vi "FirmataConstants.vi"(8 "error in":errorcluster) -> (0 "error out":errorcluster, 2 "FirmataCapabilities":T2 {"Index"."DigitalIndex" step=1 format="D%d"; "Index"."AnalogIndex" min=0.0 step=1.0 format="A%#.0g"})   [LabVIEW 2020, in "FirmataClient.lvlib"]
doc: "Repository for Firmata Protocol Constants\n- https://github.com/firmata/protocol/blob/master/protocol.md"
uses:
  FirmataClient.lvlib
  controls/PinModesListData.ctl
  controls/PinModeData.ctl
  controls/FirmataPinModes.ctl
  controls/FirmataProtocolConstants.ctl
  <vilib>/Utility/miscctls.llb/LVStringsAndValuesArrayTypeDef_U16.ctl
panel:
  in  "Reload Constant?":bool
  out "FimataProtocolConstants":T1 items=["ANALOG_IO_MESSAGE"=224, "DIGITAL_IO_MESSAGE"=144, "REPORT_ANALOG_PIN"=192, "REPORT_DIGITAL_PORT"=208, "START_SYSEX"=240, "END_SYSEX"=247, "SET_PIN_MODE"=244, "SET_DIGITAL_PIN_VALUE"=245, "PROTOCOL_VERSION"=249, "SYSTEM_RESET"=255, "SYSEX.EXTENDED_ID"=0, "SYSEX.RESERVED_USER_COMMANDs"=1, "SYSEX.ANALOG_MAPPING_QUERY"=105, "SYSEX.ANALOG_MAPPING_RESPONSE"=106, "SYSEX.CAPABILITY_QUERY"=107, "SYSEX.CAPABILITY_RESPONSE"=108, "SYSEX.PIN_STATE_QUERY"=109, "SYSEX.PIN_STATE_RESPONSE"=110, "SYSEX.REPORT_FIRMWARE"=121, "SYSEX.EXTENDED_ANALOG"=111, "SYSEX.STRING_DATA"=113, "SYSEX.REALTIME"=127, "SYSEX.NON_REALTIME"=126, "SYSEX.SAMPLING_INTERVAL"=122]
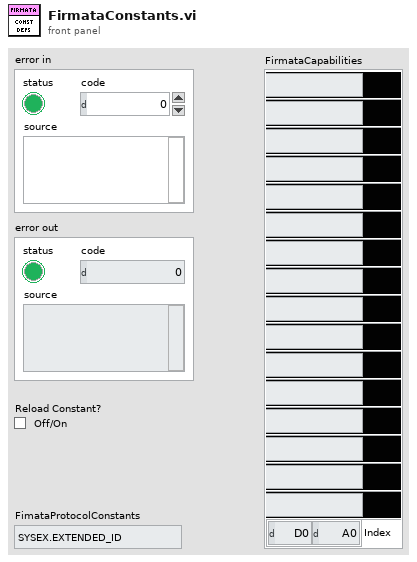
[diagram p1: front panel]
types:
  T1 = typedef "FirmataClient.lvlib/FirmataProtocolConstants.ctl" = u16
  T2 = typedef "FirmataClient.lvlib/PinModesListData.ctl" = cluster{"DigitalInputMode":T3, "DigitalOutputMode":T3, "AnalogInputMode":T3, "PWMMode":T3, "ServoMode":T3, "ShiftMode":T3, "I2CMode":T3, "OneWireMode":T3, "StepperMode":T3, "EncoderMode":T3, "SerialMode":T3, "InputPullupMode":T3, "Ext.SPIMode":T3, "Ext.SonarMode":T3, "Ext.ToneMode":T3, "Ext.DHTMode":T3, "Index":cluster{"DigitalIndex":u16, "AnalogIndex":dbl}}
  T3 = typedef "FirmataClient.lvlib/PinModeData.ctl" = cluster{"Resolution":u8, "btn":bool, "PinMode":T4}
  T4 = typedef "FirmataClient.lvlib/FirmataPinModes.ctl" = enum16{"DigitalInput", "DigitalOutput", "AnalogInput", "PWM", "Servo", "Shift", "I2C", "OneWire", "Stepper", "Encoder", "Serial", "InputPullup", "Extended.SPI", "Extended.Sonar", "Extended.Tone", "Extended.DHT"}
  T5 = typedef "LVStringsAndValuesArrayTypeDef_U16.ctl" = cluster{"String":string, "Value":u16}[]
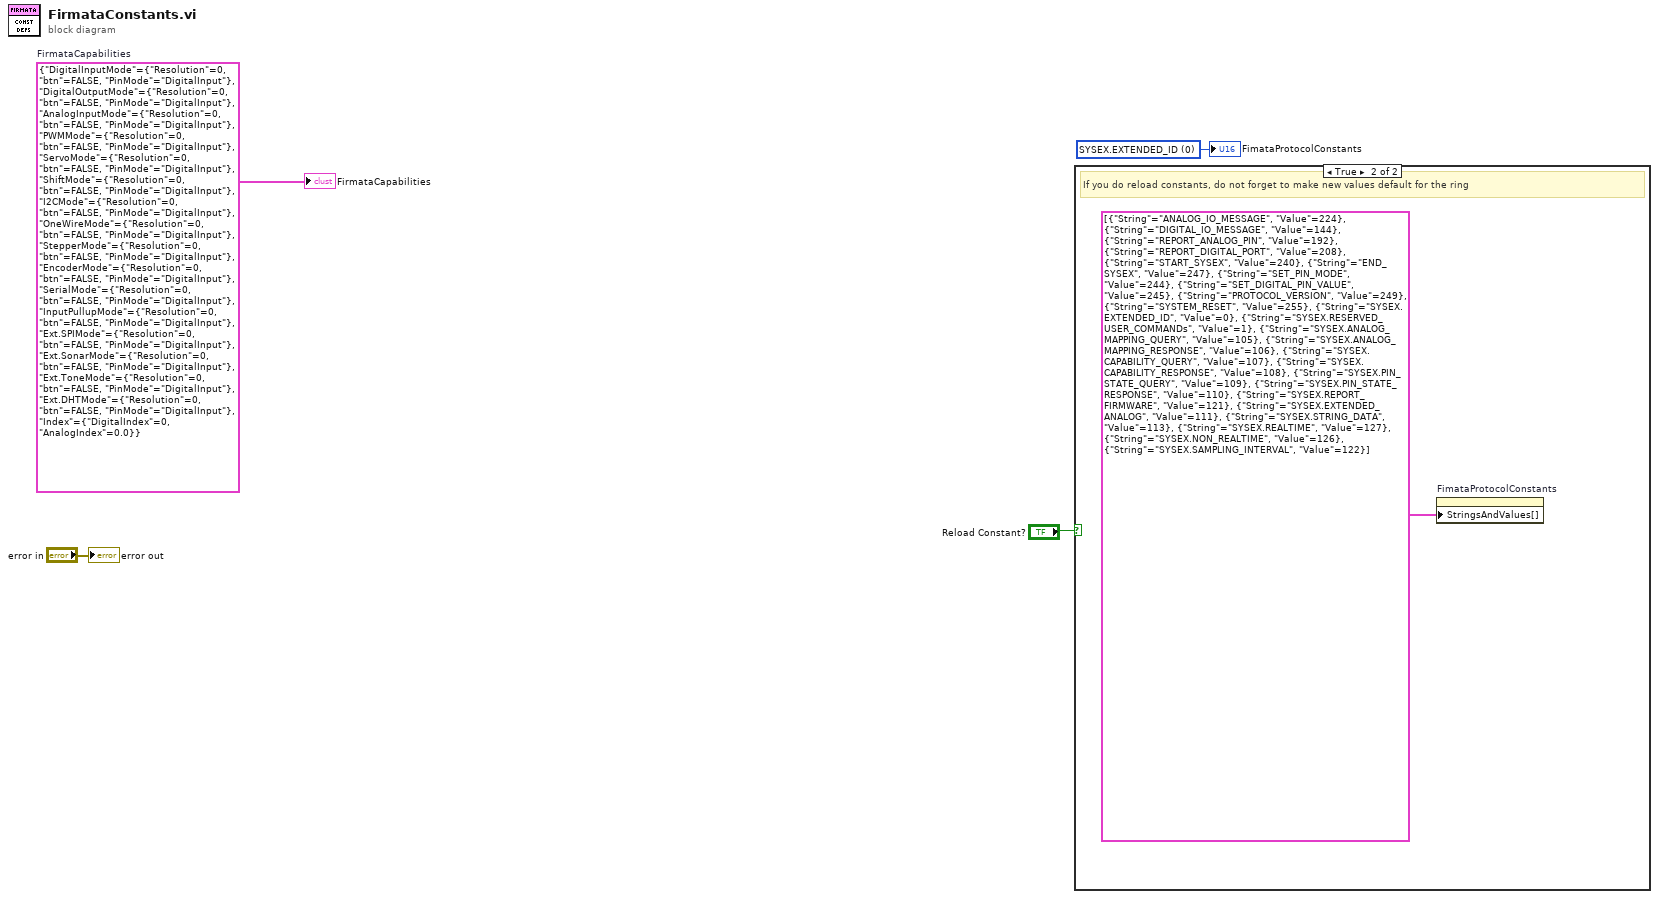
[diagram p0: block diagram]
diagram:
  w2 = T1 0 items=["ANALOG_IO_MESSAGE"=224, "DIGITAL_IO_MESSAGE"=144, "REPORT_ANALOG_PIN"=192, "REPORT_DIGITAL_PORT"=208, "START_SYSEX"=240, "END_SYSEX"=247, "SET_PIN_MODE"=244, "SET_DIGITAL_PIN_VALUE"=245, "PROTOCOL_VERSION"=249, "SYSTEM_RESET"=255, "SYSEX.EXTENDED_ID"=0, "SYSEX.RESERVED_USER_COMMANDs"=1, "SYSEX.ANALOG_MAPPING_QUERY"=105, "SYSEX.ANALOG_MAPPING_RESPONSE"=106, "SYSEX.CAPABILITY_QUERY"=107, "SYSEX.CAPABILITY_RESPONSE"=108, "SYSEX.PIN_STATE_QUERY"=109, "SYSEX.PIN_STATE_RESPONSE"=110, "SYSEX.REPORT_FIRMWARE"=121, "SYSEX.EXTENDED_ANALOG"=111, "SYSEX.STRING_DATA"=113, "SYSEX.REALTIME"=127, "SYSEX.NON_REALTIME"=126, "SYSEX.SAMPLING_INTERVAL"=122] ("FimataProtocolConstants")
  w3 = T2 {"DigitalInputMode"={"Resolution"=0, "btn"=FALSE, "PinMode"=enum."DigitalInput"}, "DigitalOutputMode"={"Resolution"=0, "btn"=FALSE, "PinMode"=enum."DigitalInput"}, "AnalogInputMode"={"Resolution"=0, "btn"=FALSE, "PinMode"=enum."DigitalInput"}, "PWMMode"={"Resolution"=0, "btn"=FALSE, "PinMode"=enum."DigitalInput"}, "ServoMode"={"Resolution"=0, "btn"=FALSE, "PinMode"=enum."DigitalInput"}, "ShiftMode"={"Resolution"=0, "btn"=FALSE, "PinMode"=enum."DigitalInput"}, "I2CMode"={"Resolution"=0, "btn"=FALSE, "PinMode"=enum."DigitalInput"}, "OneWireMode"={"Resolution"=0, "btn"=FALSE, "PinMode"=enum."DigitalInput"}, "StepperMode"={"Resolution"=0, "btn"=FALSE, "PinMode"=enum."DigitalInput"}, "EncoderMode"={"Resolution"=0, "btn"=FALSE, "PinMode"=enum."DigitalInput"}, "SerialMode"={"Resolution"=0, "btn"=FALSE, "PinMode"=enum."DigitalInput"}, "InputPullupMode"={"Resolution"=0, "btn"=FALSE, "PinMode"=enum."DigitalInput"}, "Ext.SPIMode"={"Resolution"=0, "btn"=FALSE, "PinMode"=enum."DigitalInput"}, "Ext.SonarMode"={"Resolution"=0, "btn"=FALSE, "PinMode"=enum."DigitalInput"}, "Ext.ToneMode"={"Resolution"=0, "btn"=FALSE, "PinMode"=enum."DigitalInput"}, "Ext.DHTMode"={"Resolution"=0, "btn"=FALSE, "PinMode"=enum."DigitalInput"}, "Index"={"DigitalIndex"=0, "AnalogIndex"=0.0}}  # FirmataCapabilities
  n1 = case shown="True" "Reload Constant?" {
    frame False {
    }
    frame True {
      # "If you do reload constants, do not forget to make new values default for the ring"
      n2 = property on="FimataProtocolConstants" class="Ring (strict)"("StringsAndValues[]"=T5 [{"String"="ANALOG_IO_MESSAGE", "Value"=224}, {"String"="DIGITAL_IO_MESSAGE", "Value"=144}, {"String"="REPORT_ANALOG_PIN", "Value"=192}, {"String"="REPORT_DIGITAL_PORT", "Value"=208}, {"String"="START_SYSEX", "Value"=240}, {"String"="END_SYSEX", "Value"=247}, {"String"="SET_PIN_MODE", "Value"=244}, {"String"="SET_DIGITAL_PIN_VALUE", "Value"=245}, {"String"="PROTOCOL_VERSION", "Value"=249}, {"String"="SYSTEM_RESET", "Value"=255}, {"String"="SYSEX.EXTENDED_ID", "Value"=0}, {"String"="SYSEX.RESERVED_USER_COMMANDs", "Value"=1}, {"String"="SYSEX.ANALOG_MAPPING_QUERY", "Value"=105}, {"String"="SYSEX.ANALOG_MAPPING_RESPONSE", "Value"=106}, {"String"="SYSEX.CAPABILITY_QUERY", "Value"=107}, {"String"="SYSEX.CAPABILITY_RESPONSE", "Value"=108}, {"String"="SYSEX.PIN_STATE_QUERY", "Value"=109}, {"String"="SYSEX.PIN_STATE_RESPONSE", "Value"=110}, {"String"="SYSEX.REPORT_FIRMWARE", "Value"=121}, {"String"="SYSEX.EXTENDED_ANALOG", "Value"=111}, {"String"="SYSEX.STRING_DATA", "Value"=113}, {"String"="SYSEX.REALTIME", "Value"=127}, {"String"="SYSEX.NON_REALTIME", "Value"=126}, {"String"="SYSEX.SAMPLING_INTERVAL", "Value"=122}] ("Strings And Values []")) -> ()  [unwired: 2 in, 2 out]
    }
  }
  "error out" <- "error in"
  "FirmataCapabilities" <- w3
  "FimataProtocolConstants" <- w2
